vi "Visual Table and Error Graph.vi"(10 "Measured Point":cluster{"Measured Y":dbl, "Measured X":dbl}, 11 "Set Point":cluster{"Y":dbl, "X":dbl}) -> (2 "Error Graph":cluster{dbl, dbl}, 3 "new picture":picture)   [LabVIEW 2015]
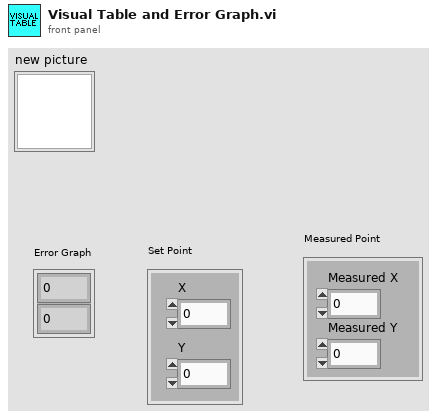
[diagram p1: front panel]
types:
  T1 = cluster{"left":i16, "top":i16, "right":i16, "bottom":i16}
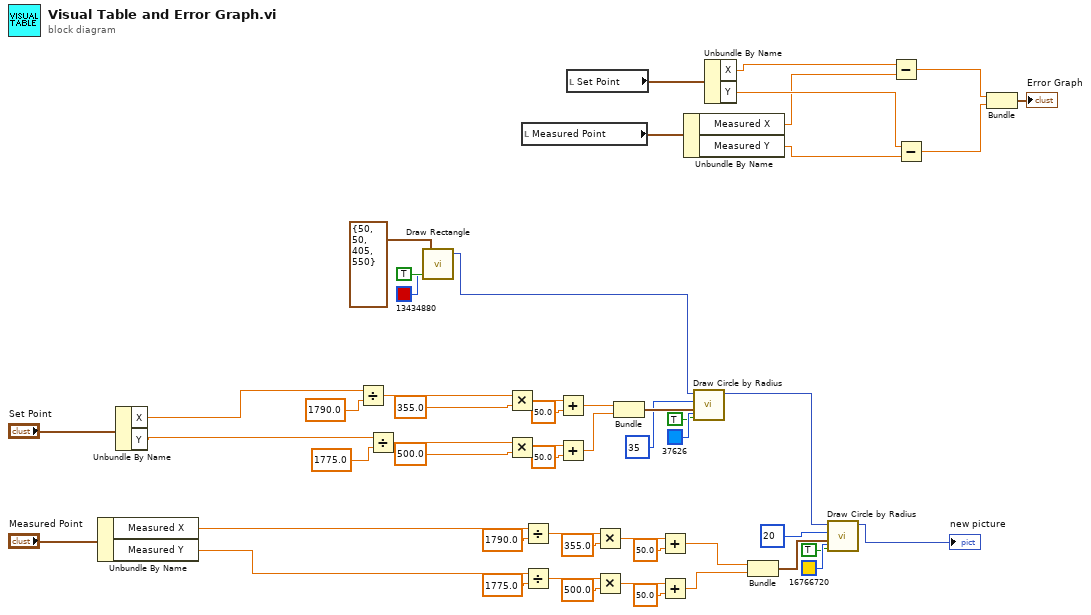
[diagram p0: block diagram]
diagram:
  n1 = Unbundle By Name("Measured Point") -> ("Measured X"=w12:dbl, "Measured Y"=w11:dbl)
  n2 = Unbundle By Name("Set Point") -> ("X"=w15:dbl, "Y"=w14:dbl)
  n3 = Divide(x=w15, y=1790.0) -> (x/y=w28:dbl)
  n4 = Divide(x=w14, y=1775.0) -> (x/y=w21:dbl)
  n5 = call <vilib>:"Draw Rectangle.vi"("rect"=T1 {"left"=50, "top"=50, "right"=405, "bottom"=550}, "fill?(F)"=TRUE, "color(black)"=u32 13434880) -> ("new picture"=w1:picture)  [unwired: 6 in]
  n6 = Multiply(x=w28, y=355.0) -> (x*y=w26:dbl)
  n7 = Multiply(x=w21, y=500.0) -> (x*y=w23:dbl)
  n8 = local read "Measured Point"() -> (w7:cluster{"Measured Y":dbl, "Measured X":dbl})
  n9 = Divide(x=w12, y=1790.0) -> (x/y=w39:dbl)
  n10 = Divide(x=w11, y=1775.0) -> (x/y=w46:dbl)
  n11 = Add(x=w26, y=50.0) -> (x+y=w51:dbl)
  n12 = Add(x=w23, y=50.0) -> (x+y=w52:dbl)
  n13 = local read "Set Point"() -> (w10:cluster{"Y":dbl, "X":dbl})
  n14 = Multiply(x=w39, y=355.0) -> (x*y=w41:dbl)
  n15 = Multiply(x=w46, y=500.0) -> (x*y=w44:dbl)
  n16 = Bundle(w51, w52) -> (w53:cluster{dbl, dbl})  [unwired: 1 in]
  n17 = Add(x=w41, y=50.0) -> (x+y=w49:dbl)
  n18 = Add(x=w44, y=50.0) -> (x+y=w48:dbl)
  n19 = Unbundle By Name(w7) -> ("Measured X"=w6:dbl, "Measured Y"=w5:dbl)
  n20 = call <vilib>:"Draw Circle by Radius.vi"("color(black)"=u32 37626, "fill?(F)"=TRUE, "pixel center"=w53, "radius"=i16 35, "picture"=w1) -> ("new picture"=w31:picture)  [unwired: 6 in]
  n21 = Unbundle By Name(w10) -> ("X"=w9:dbl, "Y"=w8:dbl)
  n22 = Bundle(w49, w48) -> (w50:cluster{dbl, dbl})  [unwired: 1 in]
  n23 = call <vilib>:"Draw Circle by Radius.vi"("color(black)"=u32 16766720, "fill?(F)"=TRUE, "pixel center"=w50, "radius"=i16 20, "picture"=w31) -> ("new picture"=→"new picture":picture)  [unwired: 6 in]
  n24 = Subtract(x=w9, y=w6) -> (x-y=w19:dbl)
  n25 = Subtract(x=w8, y=w5) -> (x-y=w18:dbl)
  n26 = Bundle(w19, w18) -> (→"Error Graph":cluster{dbl, dbl})  [unwired: 1 in]
